vi "Construct Channel List.vi"(1 "Add Comma (True)":bool=TRUE, 3 "Channel List":string) -> (0 "Channel List String":string)   [LabVIEW 2016, in "Keithley DMM6500 DAQ6500 Series.lvlib"]
doc: "Constructs Channel list for command"
uses:
  Keithley DMM6500 DAQ6500 Series.lvlib
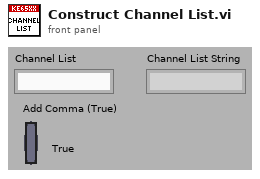
[diagram p1: front panel]
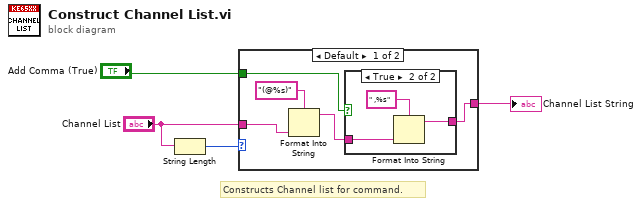
[diagram p0: block diagram]
diagram:
  # "Constructs Channel list for command."
  n1 = String Length(string="Channel List") -> (length=w3:i32)
  n2 = case shown="Default" w3 {
    tunnel: [w6 w14] -> w2
    tunnel: "Channel List" -> [w9 w14]
    tunnel: "Add Comma (True)" -> [w5 _]
    frame Default {
      n3 = Format Into String(format string="(@%s)", w9) -> (resulting string=w7:string)  [unwired: 2 in, 1 out]
      n4 = case shown="True" w5 {
        tunnel: w7 -> [w10 w12]
        tunnel: [w10 w11] -> w6
        frame False {
        }
        frame True {
          n5 = Format Into String(format string=" ,%s", w12) -> (resulting string=w11:string)  [unwired: 2 in, 1 out]
        }
      }
    }
    frame 0 {
    }
  }
  "Channel List String" <- w2
